vi "Create.vi"(8 "Error In":errorcluster, 10 "Tag":string, 11 "Square In":refnum<class "Square.lvclass">) -> (0 "Error Out":errorcluster, 3 "Square Out":refnum<class "Square.lvclass">)   [LabVIEW 2019, in "Square.lvclass"]
uses:
  Square.lvclass
  Display Element/Display Element.lvclass
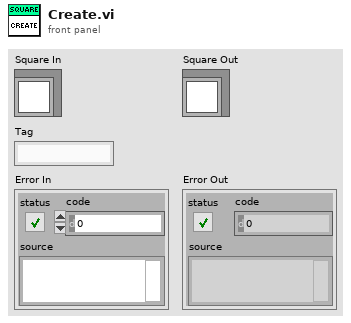
[diagram p1: front panel]
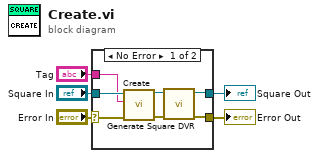
[diagram p0: block diagram]
diagram:
  n1 = case shown="No Error" "Error In" {
    selector: "Error In" -> [w12 w13]
    tunnel: [w7 w13] -> w5
    tunnel: [w6 w14] -> w4
    tunnel: "Square In" -> [w11 w14]
    tunnel: "Tag" -> [w10 _]
    frame No Error {
      n2 = call-parent "Create.vi"("Error In"=w12, "Tag"=w10, "Display Element In"=w11) -> ("Error Out"=w8:errorcluster, "Display Element"=w9:refnum<class "Square.lvclass">)  [unwired: 7 in]
      n3 = call "Generate Square DVR.vi"("Error In"=w8, "Pixel In"=w9) -> ("Error Out"=w7:errorcluster, "Pixel Out"=w6:refnum<class "Square.lvclass">)  [unwired: 8 in]
    }
    frame Error {
    }
  }
  "Square Out" <- w4
  "Error Out" <- w5
